vi "export.vi"(8 "error in (no error)":errorcluster, 10 "Shape":refnum<class "Shape.lvclass">, 11 "XMLExportVisitor in":refnum<class "XMLExportVisitor.lvclass">) -> (0 "error out":errorcluster, 2 "String":string, 3 "XMLExportVisitor out":refnum<class "XMLExportVisitor.lvclass">)   [LabVIEW 2017, in "XMLExportVisitor.lvclass"]
uses:
  XMLExportVisitor.lvclass
  C:/Users/fflores/Documents/LabVIEW-Open-Projects/LabIVEW OOP Design Patterns/Visitor Pattern/Visitor Class/Visitor.lvclass
  Shape Class/Shape.lvclass
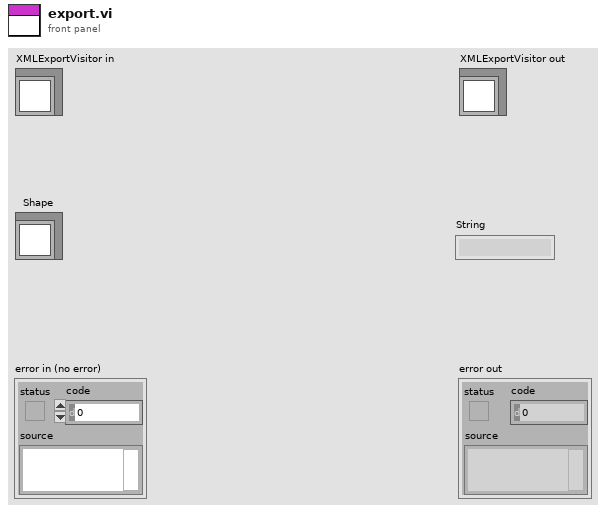
[diagram p1: front panel]
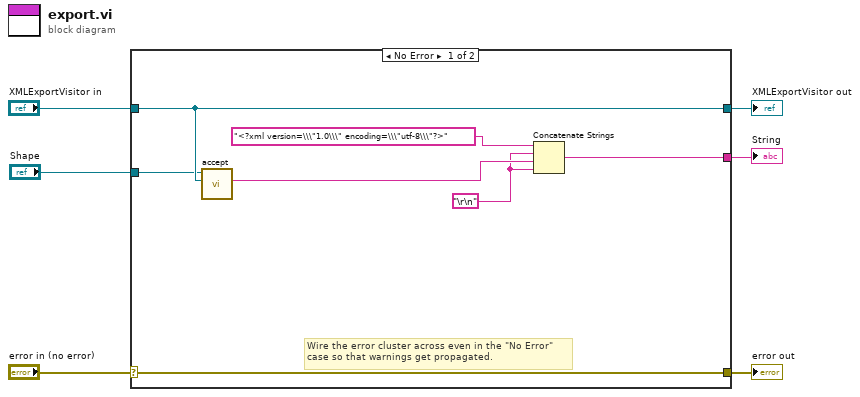
[diagram p0: block diagram]
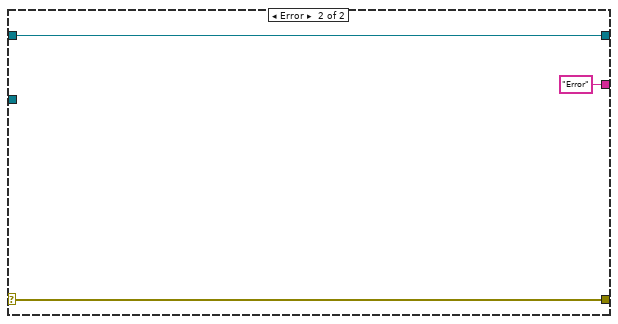
[diagram p2: hidden frame]
diagram:
  n1 = case shown="No Error" "error in (no error)" {
    selector: "error in (no error)" -> [w13 w16]
    tunnel: [w13 w16] -> w5
    tunnel: [w11 w15] -> w3
    tunnel: "XMLExportVisitor in" -> [w11 w15]
    tunnel: "Shape" -> [w10 _]
    tunnel: [w7 "Error"] -> w1
    frame No Error {
      w8 = "\r\n"
      # "Wire the error cluster across even in the \"No Error\"\ncase so that warnings get propagated."
      n2 = call-dynamic "accept.vi"("Visitor"=w11, "Shape in"=w10) -> ("String"=w9:string)  [unwired: 7 in, 2 out]
      n3 = Concatenate Strings("<?xml version=\\\"1.0\\\" encoding=\\\"utf-8\\\"?>", w8, w9, w8) -> (w7:string)
    }
    frame Error {
    }
  }
  "error out" <- w5
  "XMLExportVisitor out" <- w3
  "String" <- w1
